vi "Integration.vi"(5 "formula":string, 6 "end":dbl=1.0 format="%.2f", 7 "start":dbl format="%.2f") -> (0 "ticks":u32, 1 "error":i32, 2 "Integral of Y":dbl[](array[numeric]) format="%.2f", 3 "Y Values":dbl[](array[numeric]) format="%.2f", 4 "X Values":dbl[](array[numeric]) format="%.2f")   [LabVIEW 2020, in "NI_Gmath.lvlib"]
doc: "Calculates both the function values and the integral of a 1D function between <B>start</B> and <B>end</B>. The function is defined by a <B>formula</B>. The number of points to be calculated depends on the complexity of the given function."
uses:
  NI_Gmath.lvlib
panel:
  # "Example:\n\n start: 0.0\n end: 1.0\n formula: sin(t*t)+t"
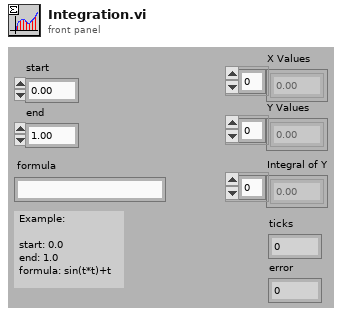
[diagram p1: front panel]
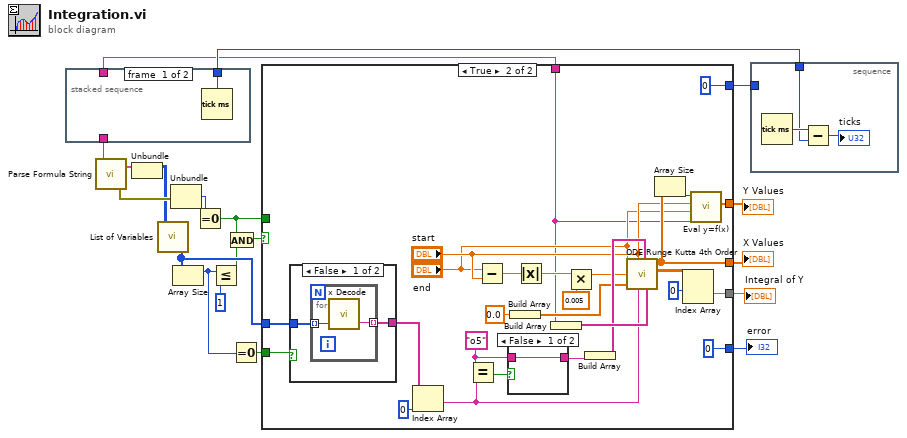
[diagram p0: block diagram]
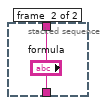
[diagram p2: hidden frame]
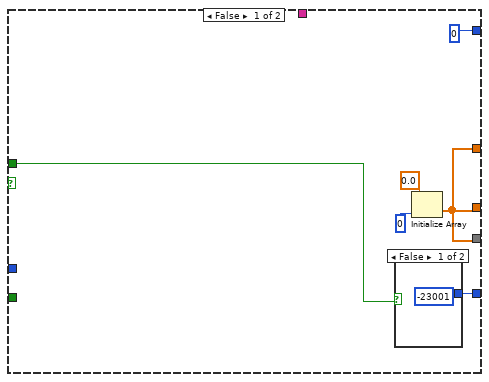
[diagram p3: hidden frame]
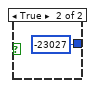
[diagram p4: hidden frame]
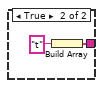
[diagram p5: hidden frame]
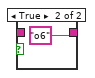
[diagram p6: hidden frame]
diagram:
  n1 = stacked-sequence {
    tunnel: [w20 _] -> w16
    tunnel: [_ "formula"] -> w2
    tunnel: [_ "formula"] -> w1
    frame #0 {
      n2 = Tick Count (ms)() -> (millisecond timer value=w20:u32)
    }
    frame #1 {
    }
  }
  n3 = call "Parse Formula String.vi"("formula"=w1) -> ("error out"=w12:errorcluster, "Parsed Formula"=w5:cluster{"Table":i32[][], "Y Values":dbl[]})  [unwired: 1 in]
  n4 = Unbundle(w5) -> ("Table"=w4:i32[][])  [unwired: 1 out]
  n5 = call "List of Variables.vi"("Table"=w4) -> ("List of variables"=w17:i32[])
  n6 = Unbundle(w12) -> ("code"=w11:i32)  [unwired: 2 out]
  n7 = Array Size(array=w17) -> (size(s)=w7:i32)
  n8 = Equal To 0?(x=w11) -> (x = 0?=w8:bool)
  n9 = Less Or Equal?(x=w7, y=1) -> (x <= y?=w9:bool)
  n10 = And(x=w8, y=w9) -> (x .and. y?=w19:bool)
  n11 = Equal To 0?(x=w7) -> (x = 0?=w6:bool)
  n12 = case shown="True" w19 {
    tunnel: w2 -> [_ w30]
    tunnel: w17 -> [_ w56]
    tunnel: [0 0] -> w15
    tunnel: [w22 w35] -> w14
    tunnel: [w22 w46] -> w13
    tunnel: [w24 0] -> w10
    tunnel: w8 -> [w23 _]
    tunnel: w6 -> [_ w41]
    tunnel: [w22 w31] -> w3
    frame False {
      n13 = case shown="False" w23 {
        tunnel: [-23001 -23027] -> w24
        frame False {
        }
        frame True {
        }
      }
      n14 = Initialize Array(0.0, 0) -> (w22:dbl[])
    }
    frame True {
      w53 = "o5"
      n15 = case shown="False" w41 {
        tunnel: [w58 w61] -> w51
        tunnel: w56 -> [w57 _]
        frame False {
          n16 = for {
            tunnel: w57 -> [w60] mode=indexing
            tunnel: [w59] -> w58 mode=indexing
            n17 = call "x Decode.vi"("number"=w60) -> ("x string"=w59:string)  [unwired: 1 in, 1 out]
          }
        }
        frame True {
          n18 = Build Array("t") -> (w61:string[])
        }
      }
      n19 = Index Array(array=w51, index=0) -> (element=w44:string)
      n20 = Equal?(x=w53, y=w44) -> (x = y?=w52:bool)
      n21 = Subtract(x="end", y="start") -> (x-y=w40:dbl)
      n22 = case shown="False" w52 {
        tunnel: w53 -> [w63 _]
        tunnel: [w63 "o6"] -> w48
        frame False {
        }
        frame True {
        }
      }
      n23 = Build Array(0.0) -> (w36:dbl[])
      n24 = Absolute Value(x=w40) -> (abs(x)=w39:dbl)
      n25 = Build Array(w30) -> (w49:string[])
      n26 = Multiply(x=w39, y=0.005) -> (x*y=w37:dbl)
      n27 = Build Array(w48) -> (w43:string[])
      n28 = call "ODE Runge Kutta 4th Order.vi"("time end"="end", "time start"="start", "h (step rate)"=w37, "X0"=w36, "time"=w44, "X (name of variables)"=w43, "F(X,t) (right sides of the ODE\nas functions of X and t)"=w49) -> ("Times"=w35:dbl[], "X Values (solution)"=w47:dbl[][])  [unwired: 2 out]
      n29 = Array Size(array=w35) -> (size(s)=w34:i32)
      n30 = Index Array(array=w47, index (col)=0) -> (element=w46:dbl[])  [unwired: 1 in]
      n31 = call "Eval y=f(x).vi"("formula"=w30, "end"="end", "start"="start", "number of points"=w34) -> ("Y Values"=w31:dbl[])  [unwired: 3 out]
    }
  }
  "error" <- w10
  "Integral of Y" <- w13
  "X Values" <- w14
  "Y Values" <- w3
  n32 = stacked-sequence {
    tunnel: w16 -> [w65]
    tunnel: w15 -> [_]
    frame #0 {
      n33 = Tick Count (ms)() -> (millisecond timer value=w66:u32)
      n34 = Subtract(x=w66, y=w65) -> (x-y=→"ticks":u32)
    }
  }
